vi "RecieveConnection.vi"() -> ()   [LabVIEW 2013, in "main.lvlib"]
uses:
  main.lvlib
panel:
  out "channel":u16
  out "remote address":string
  in  "Stop":bool
  out "data out 2":string
  out "data out":string
  out "service list":T1(array[cluster])
  out "Array 2":string[](array[string])
  out "Array":string[](array[string])
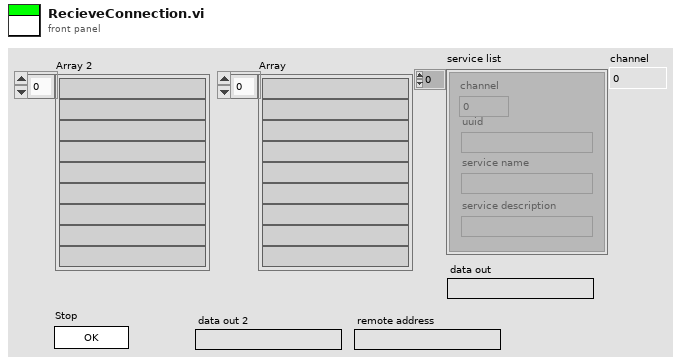
[diagram p1: front panel]
types:
  T1 = cluster{"channel":u16, "uuid":string, "service name":string, "service description":string}[]
  T2 = cluster{"Address":string, "Device Name":string}[]
  T3 = cluster{"channel":u16, "uuid":string, "service name":string, "service description":string}
  T4 = enum16{"Standard", "Buffered", "CRLF", "Immediate"}
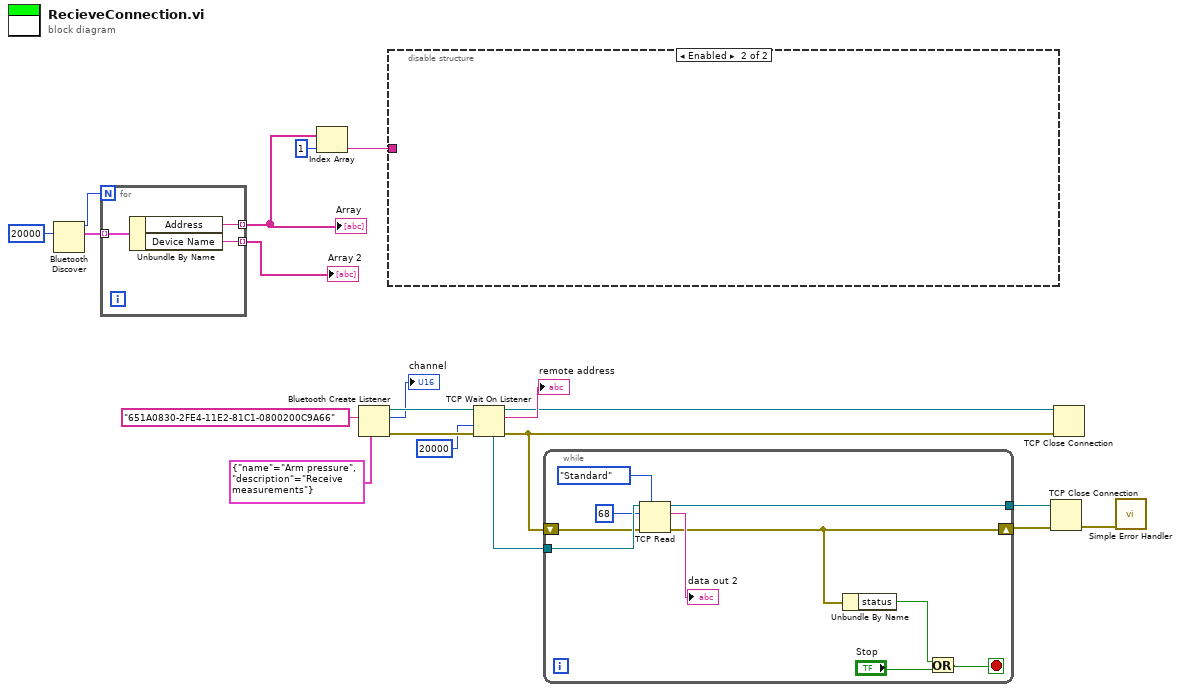
[diagram p0: block diagram]
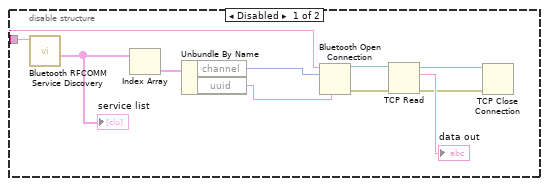
[diagram p2: hidden frame]
diagram:
  n1 = Bluetooth Discover(10:20000 ("time limit ms (10000)")) -> (2:w8:T2, 3:w9:u16)  [unwired: 1 in, 1 out]
  n2 = for {
    N: w9 -> [_]
    tunnel: w8 -> [w23] mode=indexing
    tunnel: [w22] -> w4 mode=indexing
    tunnel: [w21] -> w7 mode=indexing
    n3 = Unbundle By Name(w23) -> ("Address"=w22:string, "Device Name"=w21:string)
  }
  "Array" <- w4
  "Array 2" <- w7
  n4 = Index Array(array=w4, index=1) -> (element=w6:string)
  n5 = Bluetooth Create Listener(6:cluster{"name":string, "description":string} {"name"="Arm pressure", "description"="Receive measurements"} ("service description"), 10:"651A0830-2FE4-11E2-81C1-0800200C9A66" ("uuid")) -> (0:w17:errorcluster, 2:→"channel":u16, 3:w18:refnum<k31>)  [unwired: 2 in]
  n6 = disable-structure shown="Enabled" {
    disable-tunnel: w6 -> [w29 _]
    frame Disabled {
      n7 = call <vilib>:"Bluetooth RFCOMM Service Discovery.vi"("address in"=w29) -> ("service list"=w33:T1)  [unwired: 3 in, 3 out]
      "service list" <- w33
      n8 = Index Array(array=w33) -> (element=w32:T3)  [unwired: 1 in]
      n9 = Unbundle By Name(w32) -> ("channel"=w31:u16, "uuid"=w30:string)
      n10 = Bluetooth Open Connection(6:w30, 10:w31, 11:w29) -> (0:w27:errorcluster, 3:w28:refnum<k31>)  [unwired: 2 in]
      n11 = TCP Read(connection ID=w28, error in (no error)=w27) -> (connection ID out=w25:refnum<k31>, data out=→"data out":string, error out=w24:errorcluster)  [unwired: 3 in]
      n12 = TCP Close Connection(connection ID=w25, error in (no error)=w24) -> ()  [unwired: 1 in, 2 out]
    }
    frame Enabled {
    }
  }
  n13 = TCP Wait On Listener(8:w17, 9:20000 ("timeout ms (wait forever: -1)"), 11:w18) -> (0:w1:errorcluster, 2:→"remote address":string, 3:w2:refnum<k31>, 4:w15:refnum<k31>)  [unwired: 1 in, 1 out]
  n14 = while {
    tunnel: w15 -> [w43]
    shift-right: [w38] -> w13
    shift-left: w1 -> [w42]
    tunnel: [w37] -> w14
    stop <- w34 stop-if-true
    n15 = TCP Read(connection ID=w43, bytes to read=68, error in (no error)=w42, 7:T4."Standard" ("mode (standard)")) -> (connection ID out=w37:refnum<k31>, data out=→"data out 2":string, error out=w38:errorcluster)  [unwired: 1 in]
    n16 = Unbundle By Name(w38) -> ("status"=w35:bool)
    n17 = Or(x=w35, y="Stop") -> (x .or. y?=w34:bool)
  }
  n18 = TCP Close Connection(connection ID=w14, error in (no error)=w13) -> (error out=w12:errorcluster)  [unwired: 1 in, 1 out]
  n19 = TCP Close Connection(connection ID=w2, error in (no error)=w1) -> ()  [unwired: 1 in, 2 out]
  n20 = call <vilib>:"Simple Error Handler.vi"("error in (no error)"=w12) -> ()  [unwired: 4 in, 5 out]
